vi "Initialise RW Task.vi"(8 "error in":errorcluster) -> (0 "error out":errorcluster, 3 "R/W":refnum<k21> caption="task out")   [LabVIEW 2021, in "IO.lvclass"]
uses:
  IO.lvclass
  <vilib>/DAQmx/create/channels.llb/DAQmx Create Channel (DI-Digital Input).vi
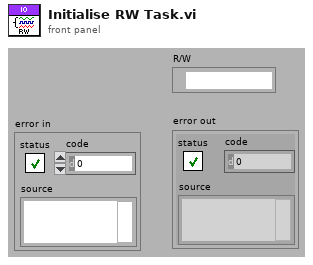
[diagram p1: front panel]
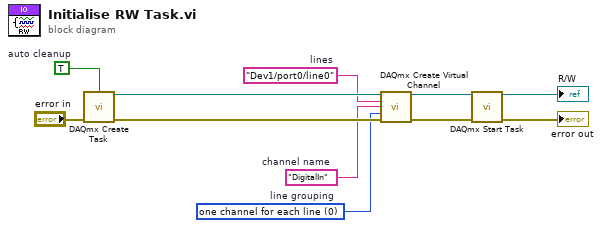
[diagram p0: block diagram]
diagram:
  w6 = 0 items=["one channel for each line", "one channel for all lines"]  # line grouping
  w5 = "DigitalIn"  # channel name
  w7 = "Dev1/port0/line0"  # lines
  w9 = TRUE  # auto cleanup
  n1 = call <vilib>:"DAQmx Create Task.vi"("auto cleanup"=w9, "error in"="error in") -> ("task out"=w8:refnum<k21>, "error out"=w10:errorcluster)  [unwired: 12 in]
  n2 = call-poly <vilib>:"DAQmx Create Virtual Channel.vi"("task in"=w8, "lines"=w7, "name to assign"=w5, "line grouping"=w6, "error in"=w10) -> ("task out"=w4:refnum<k21>, "error out"=w3:errorcluster)  [unwired: 9 in]
  n3 = call <vilib>:"DAQmx Start Task.vi"("task/channels in"=w4, "error in"=w3) -> ("task out"=→"R/W":refnum<k21>, "error out"=→"error out":errorcluster)  [unwired: 12 in]
